vi "Global 1.vi"() -> ()   [LabVIEW 2019]
uses:
  Devices/NI Board/cDAQ-9221 AI/Set_NIAI.ctl
  Devices/NI Board/cDAQ-9476 DO/cnt_Relay.ctl
  Test Mode.ctl
panel:
  out "ETime 작동대기":dbl
  in  "시험모드 선택 2":refnum<vi>
  out "Elapsed Time sum":dbl
  in  "Operation Status 2":refnum<vi>
  in  "작동시간(초)":refnum<vi>
  out "스위칭 시간":dbl
  out "Elapsed Time 작동":dbl
  out "Elapsed Time 미작동":dbl
  out "작동회수":i32
  out "950Trigger":i32
  out "data_relay":bool[](array[boolean])
  in  "read_dl950 2":string
  out "T2":dbl
  out "T1":dbl
  in  "시험 모드":T1
  out "dt(ms)_finish":u32
  out "dt(ms)_hw":u32
  out "da950_array":dbl[](array[numeric])
  in  "query delay":u32=200
  out "query done?":bool
  in  "read_dl950":string
  in  "Relay":cluster{"Relay":T2, "Boolean":bool}
  in  "lines_do":tag
  out "data":waveform(dbl)[](graph) caption="data_wave"
  out "close_ai":bool
  in  "Property_AI":T3={"input terminal"=10083, "minimum value"=-60.0, "maximum value"=60.0, "number of samples"=1000, "rate"=10000.0, "sample mode"=10123, "physical channels"=""} {"sample mode" items=["Finite Samples"=10178, "Continuous Samples"=10123, "Hardware Timed Single Point"=12522]; "rate" format="%0.2f"; "maximum value" format="%^.2e"; "minimum value" format="%^.2e"; "input terminal" items=["default"=-1, "RSE"=10083, "NRSE"=10078, "Differential"=10106, "Pseudodifferential"=12529]}
  in  "String":string
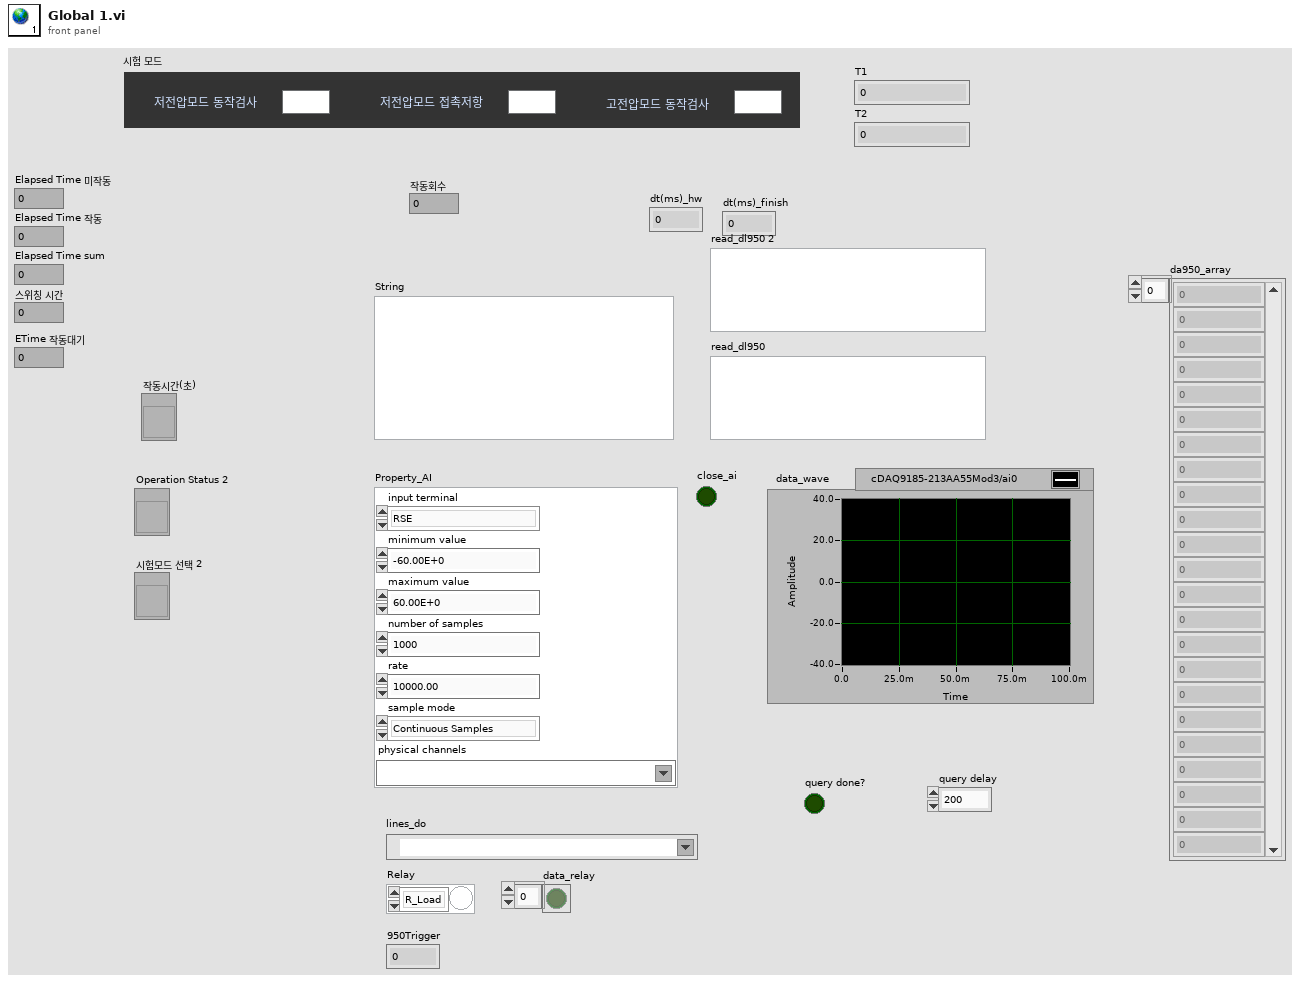
[diagram p1: front panel]
types:
  T1 = typedef "Test Mode.ctl" = enum32{"저항부하", "캐패시터부하", "B수명 - 1", "B수명 - 2", "B수명 - 3", "저전압모드 동작검사", "저전압모드 접촉저항", "고전압모드 동작검사"}
  T2 = typedef "cnt_Relay.ctl" = enum32{"R_Load", "R_out1", "R_out2", "R_out3", "R_out4", "R_out5", "R_out6", "R8", "R9", "R10", "R11", "R12", "R13", "R14", "R15", "R16", "R_in1", "R_in2", "R_in3", "R_in4", "R_in5", "R_in6", "R23", "R24", "R25", "R26", "R27", "R_red", "R_yellow", "R_green", "R_buz", "R_purple"}
  T3 = typedef "Set_NIAI.ctl" = cluster{"input terminal":i32, "minimum value":dbl, "maximum value":dbl, "number of samples":i32, "rate":dbl, "sample mode":i32, "physical channels":tag}
diagram:
